vi "GoGalvo.vi"(1 "error in":errorcluster, 2 "Galvo-resource out":T1) -> (0 "error out":errorcluster)   [LabVIEW 2011]
uses:
  SIAM/SIAM-send.ctl
panel:
  out "read buffer":string
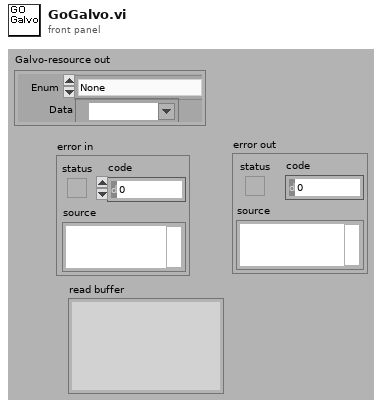
[diagram p1: front panel]
types:
  T1 = cluster{"Enum":enum16{"None", "DSP-on serial port", "Analog out", "SIAM-withDSiam"}, "Data":refnum<k21>}
  T2 = enum16{"None", "DSP-on serial port", "Analog out", "SIAM-withDSiam"}
  T3 = typedef "SIAM-send.ctl" = enum16{"validID", "storeID", "enable", "rundirect", "sendlist", "run", "stop", "readRegister", "sendValue", "storeStatus"}
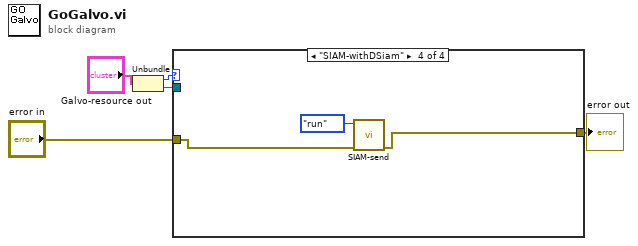
[diagram p0: block diagram]
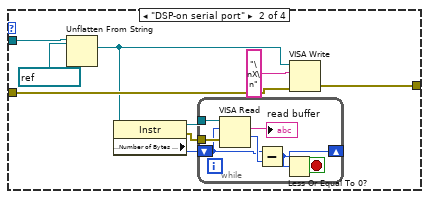
[diagram p3: hidden frame]
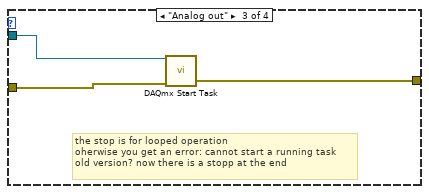
[diagram p4: hidden frame]
diagram:
  n1 = Unbundle("Galvo-resource out") -> ("Enum"=w2:T2, "Data"=w1:refnum<k21>)
  n2 = case shown="\"SIAM-withDSiam\"" w2 {
    tunnel: "error in" -> [w6 w12 w24 w28]
    tunnel: [w6 w11 w25 w27] -> w4
    tunnel: w1 -> [_ w9 w23 _]
    frame "None", Default {
    }
    frame "DSP-on serial port" {
      n3 = Unflatten From String(type=refnum<visa-resource-name> "COM1" ("DSP resource name out"), binary string=w9) -> (value=w7:refnum<visa-resource-name>)  [unwired: 1 in, 4 out]
      n4 = property class="Instr"(reference=w7) -> (reference out=w13:refnum<visa-resource-name>, error out=w14:errorcluster, "Serial Settings:Number of Bytes at Serial Port"=w15:u32)  [unwired: 1 in]
      n5 = while {
        tunnel: w14 -> [w22]
        tunnel: w13 -> [w21]
        shift-right: [w17] -> _
        shift-left: w15 -> [w18]
        stop <- w16 stop-if-true
        n6 = VISA Read(VISA resource name=w21, byte count=w18, error in (no error)=w22) -> (read buffer=→"read buffer":string, return count=w19:u32)  [unwired: 2 out]
        n7 = Subtract(x=w18, y=w19) -> (x-y=w17:u32)
        n8 = Less Or Equal To 0?(x=w17) -> (x <= 0?=w16:bool)
      }
      n9 = VISA Write(VISA resource name=w7, write buffer="\nX\n", error in (no error)=w12) -> (error out=w11:errorcluster)  [unwired: 2 out]
    }
    frame "Analog out" {
      # "the stop is for looped operation\noherwise you get an error: cannot start a running task\nold version? now there is a stopp at the end"
      n10 = call <vilib>:"DAQmx Start Task.vi"("task/channels in"=w23, "error in"=w24) -> ("error out"=w25:errorcluster)  [unwired: 13 out]
    }
    frame "SIAM-withDSiam" {
      n11 = call "SIAM-send.vi"("error in (no error)"=w28, "command"=SIAM-send."run") -> ("error out"=w27:errorcluster)  [unwired: 8 in, 1 out]
    }
  }
  "error out" <- w4
